vi "dotproduct5elemi32.vi"(1 "Array 2":i32[](array[numeric])=[0, 0, 0, 0, 0], 2 "Array":i32[](array[numeric])=[0, 0, 0, 0, 0]) -> (0 "result":i32)   [LabVIEW 2010]
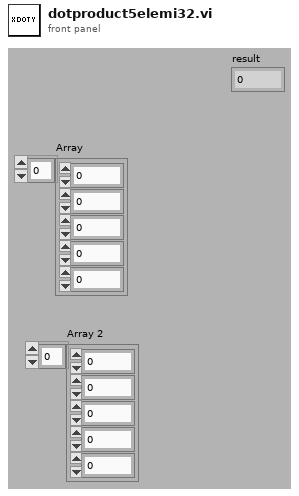
[diagram p1: front panel]
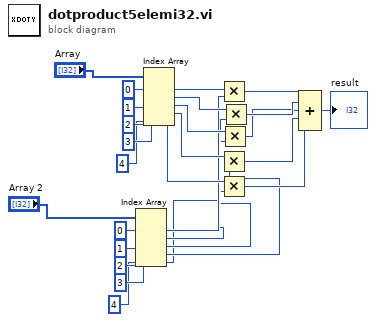
[diagram p0: block diagram]
diagram:
  n1 = Index Array(array="Array 2", index #1=0 ("index"), index #2=1 ("index"), index #3=2 ("index"), index #4=3 ("index"), index #5=4 ("index")) -> (element #1=w6:i32, element #2=w5:i32, element #3=w4:i32, element #4=w3:i32, element #5=w2:i32)
  n2 = Index Array(array="Array", index #1=0 ("index"), index #2=1 ("index"), index #3=2 ("index"), index #4=3 ("index"), index #5=4 ("index")) -> (element #1=w16:i32, element #2=w15:i32, element #3=w14:i32, element #4=w13:i32, element #5=w12:i32)
  n3 = Multiply(x=w16, y=w6) -> (x*y=w11:i32)
  n4 = Multiply(x=w13, y=w3) -> (x*y=w8:i32)
  n5 = Multiply(x=w12, y=w2) -> (x*y=w7:i32)
  n6 = Multiply(x=w14, y=w4) -> (x*y=w9:i32)
  n7 = Multiply(x=w15, y=w5) -> (x*y=w10:i32)
  n8 = Compound Arithmetic op=ADD(w11, w10, w9, w8, w7) -> (→"result":i32)
